vi "Master Program.vi"() -> ()   [LabVIEW 2017]
uses:
  <vilib>/Math Plots/3D Math Plots/3D Scatter/3D Scatter XCtrl/3D Scatter.xctl
  <vilib>/Math Plots/3D Math Plots/3D Comet/3D Comet XCtrl/3D Comet.xctl
  <vilib>/Math Plots/3D Math Plots/3D Surface/3D Surface XCtrl/3D Surface.xctl
  <vilib>/Instr/_visa.llb/VISA Flush IO Buffer Mask.ctl
  Globals.vi
  <vilib>/Instr/_visa.llb/VISA Configure Serial Port (Instr).vi
  <vilib>/Math Plots/3D Math Plots/3D Scatter/3D Scatter Datatype/Public/Plot Helper (Vector).vi
  <vilib>/Math Plots/3D Math Plots/3D Comet/3D Comet Datatype/Public/Plot Helper (Vector).vi
  <vilib>/Utility/file.llb/Read Delimited Spreadsheet (DBL).vi
  <vilib>/Utility/cursorutil.llb/Set Cursor (Icon Pict).vi
  <vilib>/Math Plots/3D Math Plots/3D Comet/3D Comet Datatype/3D Comet Datatype.lvclass
  <vilib>/Math Plots/3D Math Plots/3D Scatter/3D Scatter Datatype/3D Scatter Datatype.lvclass
  <vilib>/FTP/NI_FTP.lvlib
panel:
  out "error out 6":errorcluster caption="error out"
  out "error out 5":errorcluster
  out "file error":errorcluster
  out "error out 4":errorcluster
  out "state":dbl
  out "VISA resource name out":refnum<visa-resource-name>
  out "error out 3":errorcluster caption="error out"
  out "error out 2":errorcluster
  out "error out":errorcluster
  out "Message Window":string
  out "Data load indicator":bool
  in  "stop":bool
  in  "Close Figures":bool
  out "Load":string
  out "NX path":path caption="selected path"
  in  "Tab Control":T1(tab)
  in  "Open Webcam":bool
  in  "Form Type":u16(ring) items=["Pyramid", "NX Pattern"]
  in  "Save":bool
  out "Calculated Depth":dbl
  in  "vangle":dbl
  in  "overlap":dbl
  in  "increment":dbl
  in  "width":dbl
  in  "layers":dbl
  in  "height":dbl
  in  "Min_dist":dbl
  out "3D Scatter 2":refnum<class "3D Plot Datatype.lvclass">[](xcontrol)
  out "3D Comet":refnum<class "3D Plot Datatype.lvclass">[](xcontrol)
  in  "refresh":bool
  in  "interpolate":bool
  in  "Upload Path":bool
  in  "z offset":dbl
  in  "y offset":dbl
  in  "x offset":dbl
  in  "Min_dist initial":dbl
  in  "height initial":dbl
  in  "layers initial":dbl
  in  "width initial":dbl
  in  "increment initial":dbl
  in  "overlap initial":dbl
  in  "vangle initial":dbl
  out "Calculated Depth initial":dbl
  in  "Save Initial":bool
  out "3D Comet 2":refnum<class "3D Plot Datatype.lvclass">[](xcontrol)
  in  "Spin Graph":dbl(knob) min=-2.0 max=2.0 step=0.25 scale=-2.0..2.0
  out "Normalized Error":dbl
  in  "Plot":bool
  in  "Figure":bool
  in  "Matlab Plot":u16(ring) items=["Reference", "Initial Form Path", "Measured Data", "Error vs. Iteration", "Error vs. Command", "Error Surface", "Current Correction Path", "Error vs. Translation", "Custom"]
  out "3D Comet 3":refnum<class "3D Plot Datatype.lvclass">[](xcontrol)
  out "3D Surface":refnum<class "3D Plot Datatype.lvclass">[](xcontrol)
  out "Correction #":dbl
  in  "Save Correction":bool
  in  "Correction Factor K":dbl(slide) min=0.0 max=1.0 step=0.01 scale=0.0..1.0
  in  "Load Final Data":bool
  in  "Load Initial":bool
  in  "Graph Select":u16(ring) items=["Error Plot", "Measured Data", "Path Plot", "Reference"]
  in  "Upload Path":bool
  in  "Graph Format Code":string
  in  "Stop Robot":bool
  out "Standby":bool=TRUE
  in  "Start Robot":bool
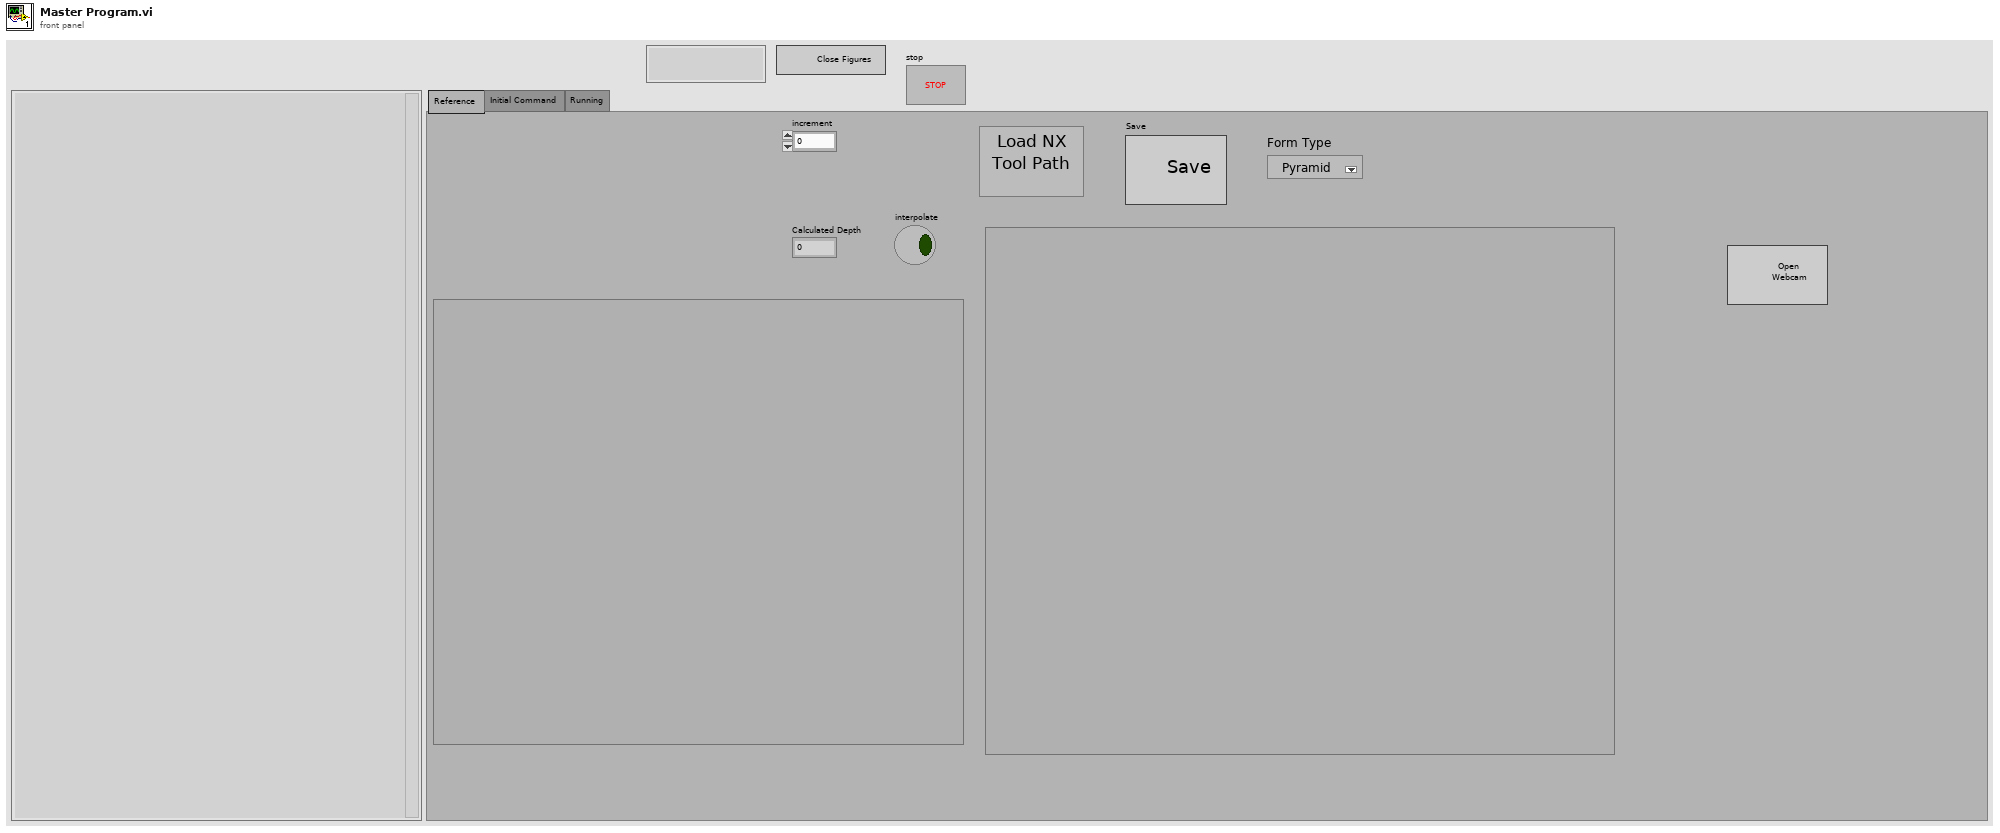
[diagram p1: front panel]
types:
  T1 = enum32{"Reference ", "Initial Command", "Running"}
  T2 = cluster{"x shift":dbl, "y shift":dbl, "z shift":dbl, "Theta x":dbl, "Theta y":dbl}
  T3 = cluster{"increment":dbl, "vangle":dbl, "overlap":dbl, "width":dbl, "height":dbl, "layers":dbl, "min_dist":dbl}
  T4 = cluster{"increment initial":dbl, "vangle initial":dbl, "overlap initial":dbl, "width initial":dbl, "height initial":dbl, "layers initial":dbl}
  T5 = typedef "VISA Flush IO Buffer Mask.ctl" = u16
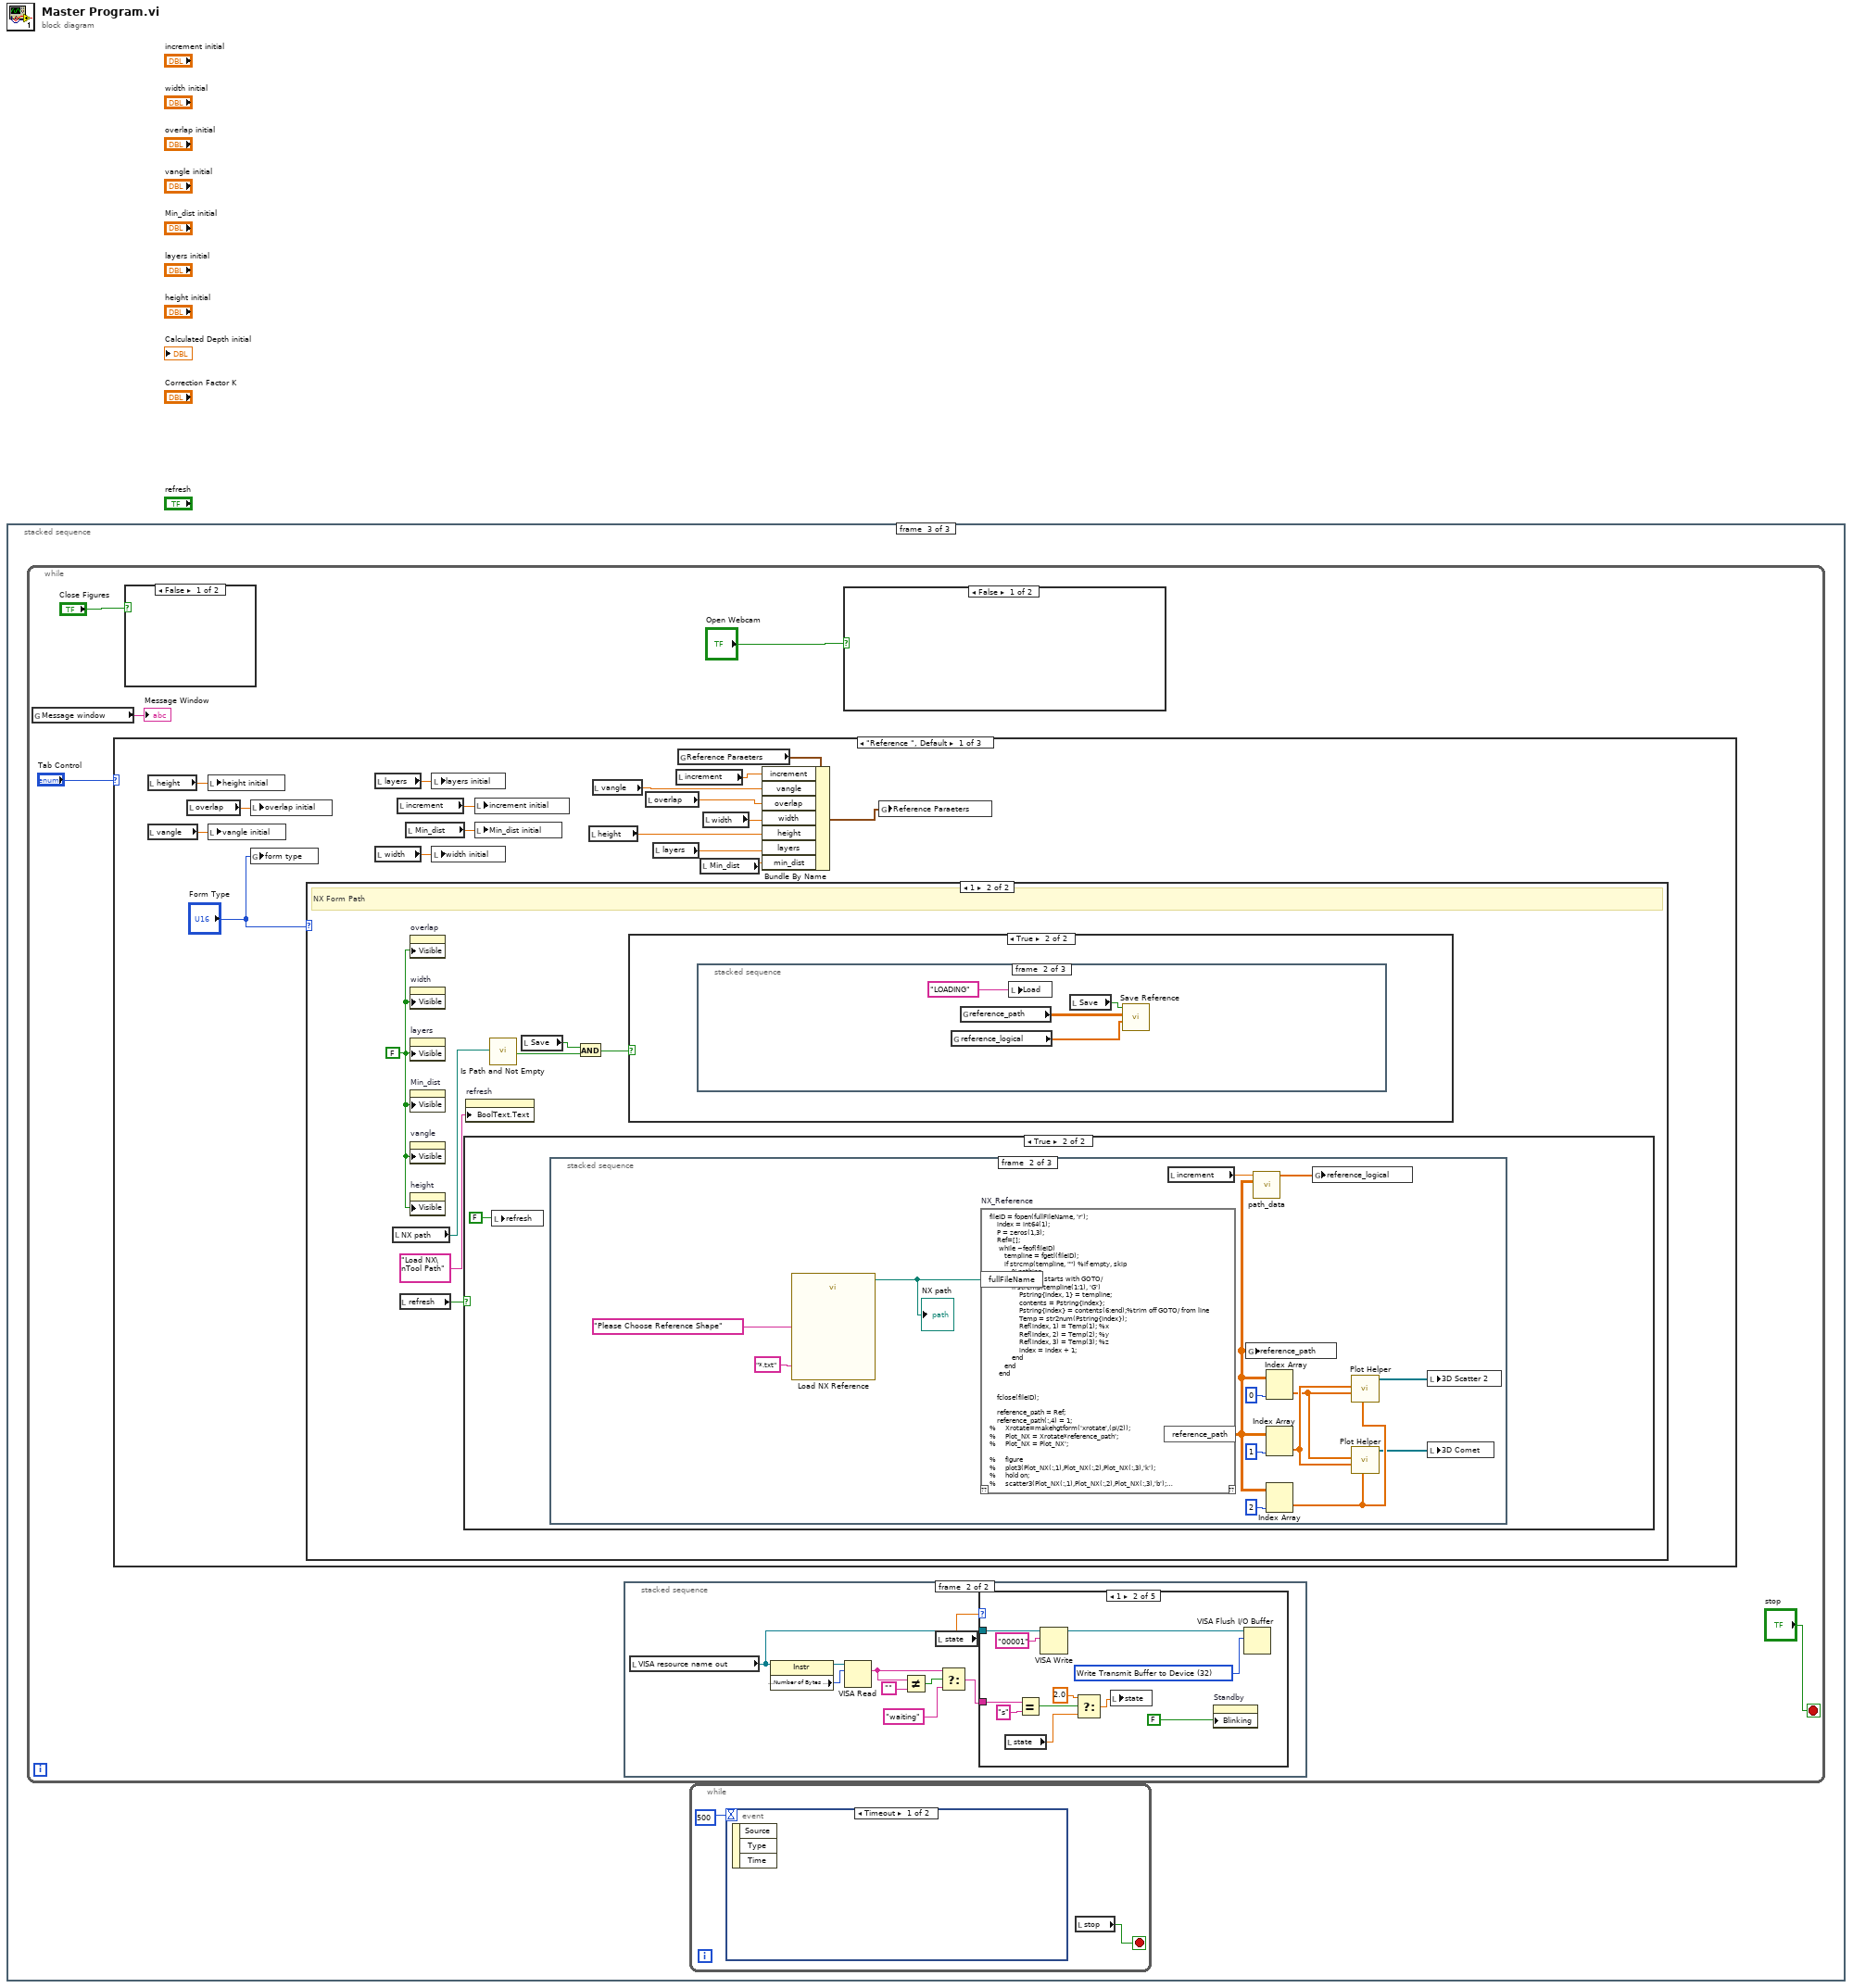
[diagram p0: block diagram]
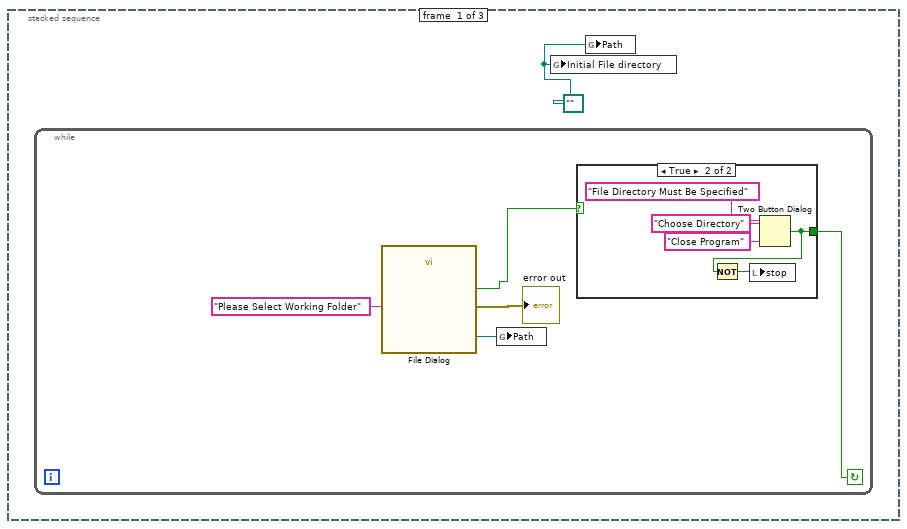
[diagram p2: hidden frame]
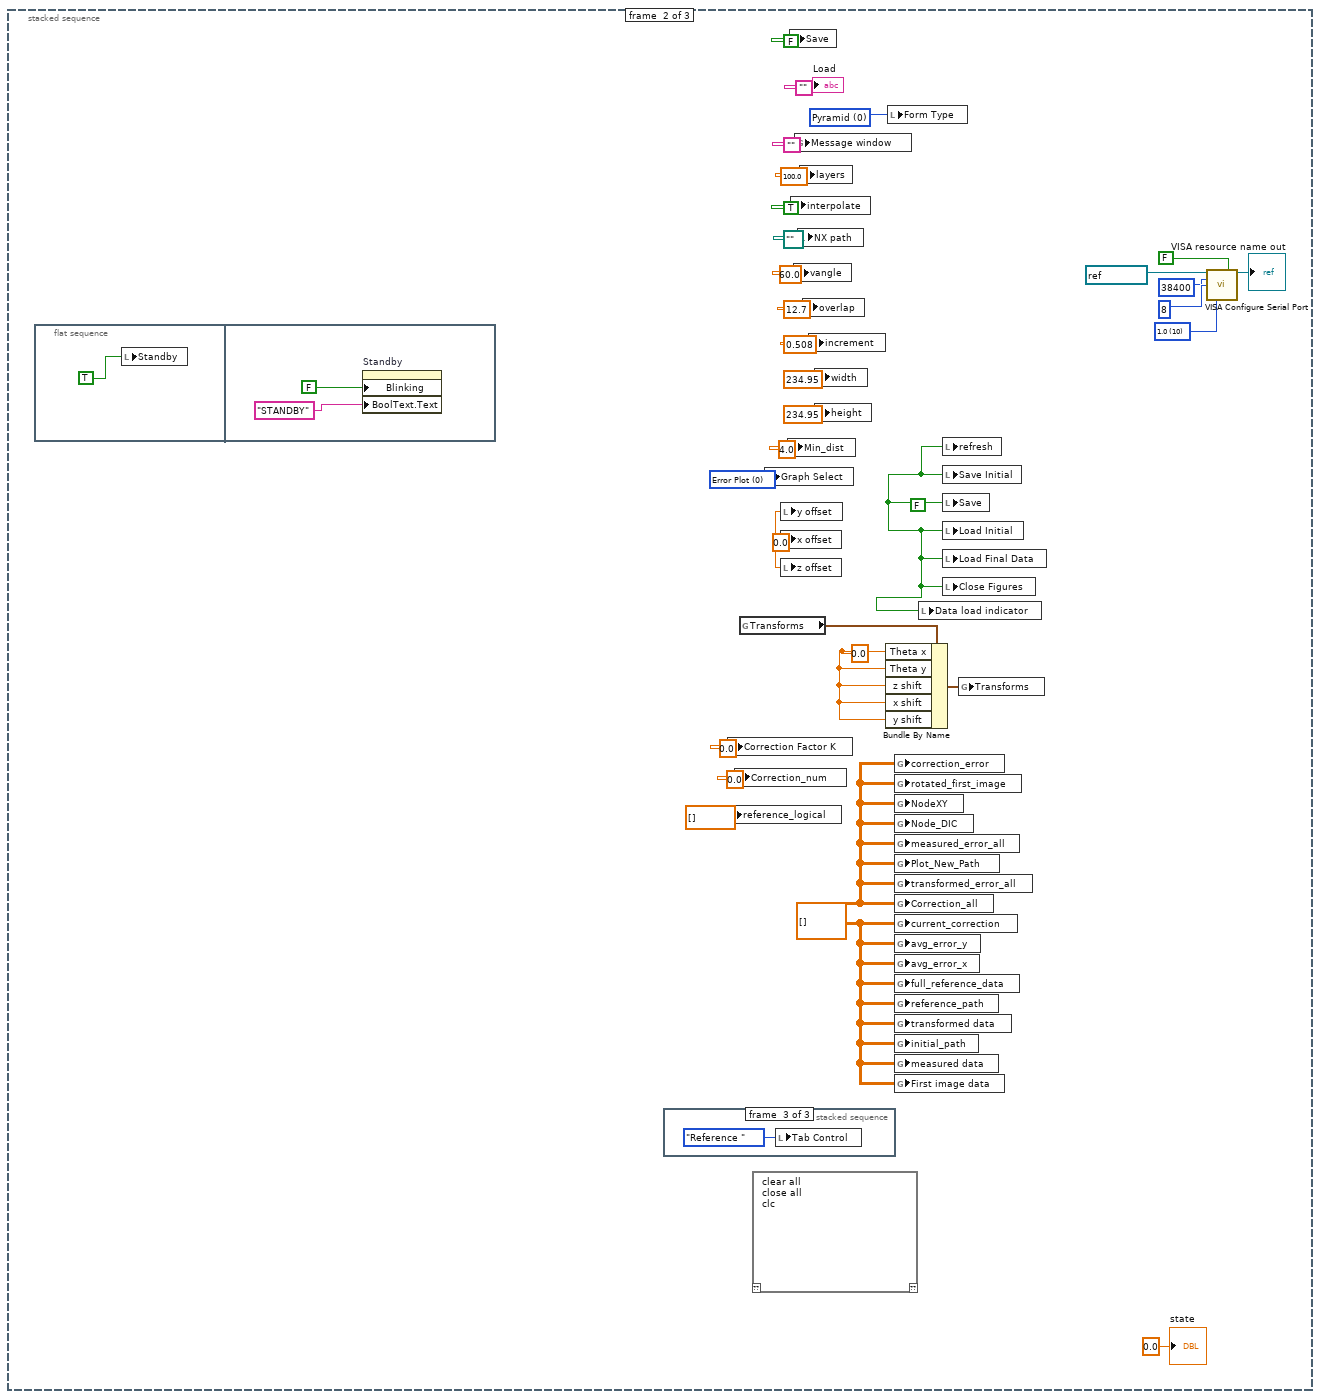
[diagram p4: hidden frame]
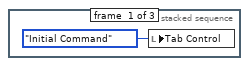
[diagram p5: hidden frame]
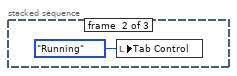
[diagram p6: hidden frame]
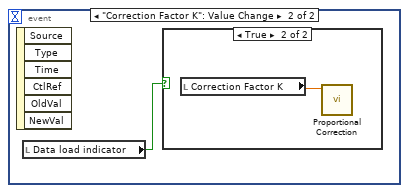
[diagram p7: hidden frame]
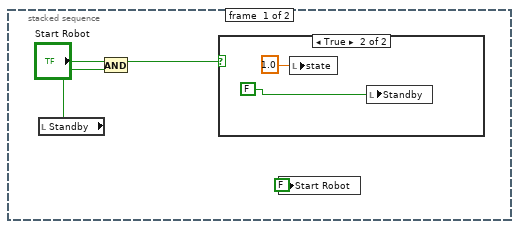
[diagram p9: hidden frame]
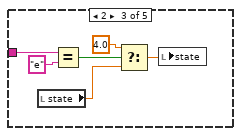
[diagram p12: hidden frame]
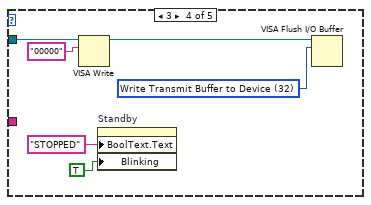
[diagram p13: hidden frame]
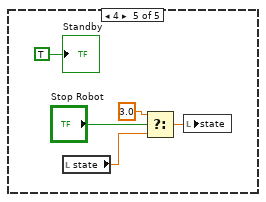
[diagram p14: hidden frame]
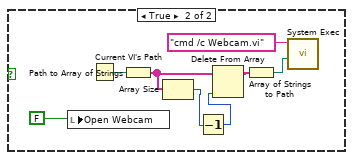
[diagram p15: hidden frame]
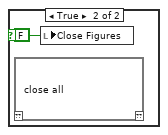
[diagram p16: hidden frame]
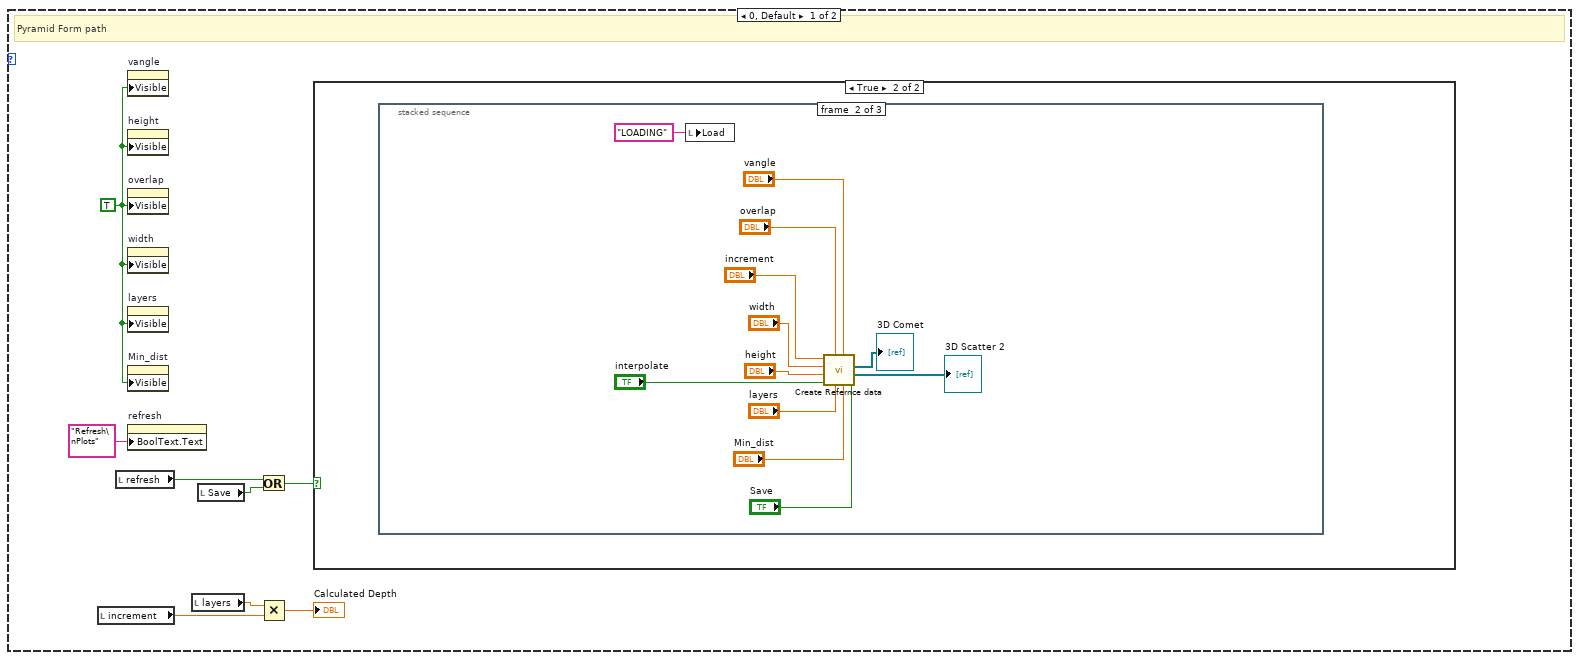
[diagram p17: hidden frame]
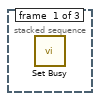
[diagram p19: hidden frame]
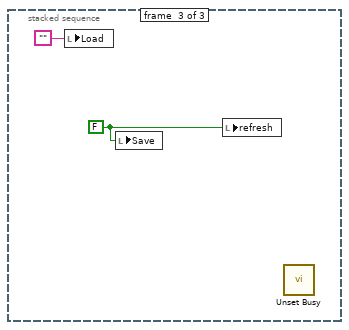
[diagram p20: hidden frame]
diagram:
  n1 = stacked-sequence {
    frame #0 {
      w1 = path "" ("Initial File directory")
      n2 = while {
        stop <- w2 continue-if-true
        n3 = call "File Dialog"("prompt"="Please Select Working Folder") -> ("selected path"=w4:path, "cancelled"=w3:bool, "error out"=→"error out":errorcluster)  [unwired: 11 in, 1 out]
        n4 = global write "Globals.vi" "Path"(w4) -> ()
        n5 = case shown="True" w3 {
          selector: w3 -> [w7 _]
          tunnel: [w7 w8] -> w2
          frame False {
          }
          frame True {
            n6 = Two Button Dialog(message="File Directory Must Be Specified", 1:"Close Program" ("F button name (\"Cancel\")"), 2:"Choose Directory" ("T button name (\"OK\")")) -> (T button?=w8:bool)
            n7 = Not(x=w8) -> (.not. x?=w9:bool)
            n8 = local write "stop"(w9) -> ()
          }
        }
      }
      n9 = global write "Globals.vi" "Initial File directory"(w1) -> ()
      n10 = global write "Globals.vi" "Path"(w1) -> ()
    }
    frame #1 {
      w16 = u16 10 items=["1.0"=10, "1.5"=15, "2.0"=20] ("stop bits (10: 1 bit)")
      w20 = u16 0 items=["Error Plot", "Measured Data", "Path Plot", "Reference"] ("Graph Select")
      w21 = dbl[][] []
      w25 = FALSE ("refresh")
      w26 = 0.0 ("z offset")
      w27 = 0.0
      w31 = u16 0 items=["Pyramid", "NX Pattern"] ("Form Type")
      n11 = flat-sequence {
        frame #0 {
          n12 = local write "Standby"(TRUE ("Standby")) -> ()
        }
        frame #1 {
          n13 = property on="Standby" class="Bool (strict)"("Blinking"=FALSE, "BoolText.Text"="STANDBY" ("Boolean Text.Text")) -> ()  [unwired: 2 in, 2 out]
        }
      }
      n14 = stacked-sequence {
        frame #0 {
          n15 = local write "Tab Control"(T1."Initial Command" ("Tab Control")) -> ()
        }
        frame #1 {
          n16 = local write "Tab Control"(T1."Running" ("Tab Control")) -> ()
        }
        frame #2 {
          n17 = local write "Tab Control"(T1."Reference " ("Tab Control")) -> ()
        }
      }
      n18 = global write "Globals.vi" "reference_logical"(dbl[] []) -> ()
      n19 = local write "Correction Factor K"(0.0 ("Correction Factor K")) -> ()
      n20 = global write "Globals.vi" "Correction_num"(0.0 ("Correction_num")) -> ()
      n21 = global read "Globals.vi" "Transforms"() -> (w29:T2)
      n22 = script code="clear all\nclose all\nclc"() -> ()  [unwired: 1 in, 1 out]
      n23 = local write "Graph Select"(w20) -> ()
      n24 = local write "y offset"(w26) -> ()
      n25 = local write "x offset"(w26) -> ()
      n26 = local write "z offset"(w26) -> ()
      n27 = local write "Min_dist"(4.0 ("vangle")) -> ()
      n28 = local write "Save"(FALSE ("Save Button")) -> ()
      n29 = local write "interpolate"(TRUE ("Interpolate")) -> ()
      n30 = local write "vangle"(60.0 ("vangle")) -> ()
      n31 = global write "Globals.vi" "Message window"("") -> ()
      n32 = local write "NX path"(path "" ("y")) -> ()
      n33 = local write "layers"(100.0 ("vangle")) -> ()
      n34 = local write "overlap"(12.7 ("vangle")) -> ()
      n35 = local write "increment"(0.508 ("vangle")) -> ()
      n36 = local write "width"(234.95 ("vangle")) -> ()
      n37 = local write "height"(234.95 ("vangle")) -> ()
      n38 = Bundle By Name(cluster=w29, "Theta x"=w27, "Theta y"=w27, "z shift"=w27, "x shift"=w27, "y shift"=w27) -> (w28:T2)
      n39 = local write "Form Type"(w31) -> ()
      n40 = global write "Globals.vi" "correction_error"(w21) -> ()
      n41 = global write "Globals.vi" "rotated_first_image"(w21) -> ()
      n42 = global write "Globals.vi" "NodeXY"(w21) -> ()
      n43 = global write "Globals.vi" "Node_DIC"(w21) -> ()
      n44 = global write "Globals.vi" "measured_error_all"(w21) -> ()
      n45 = global write "Globals.vi" "Plot_New_Path"(w21) -> ()
      n46 = global write "Globals.vi" "transformed_error_all"(w21) -> ()
      n47 = global write "Globals.vi" "Correction_all"(w21) -> ()
      n48 = global write "Globals.vi" "current_correction"(w21) -> ()
      n49 = global write "Globals.vi" "avg_error_y"(w21) -> ()
      n50 = global write "Globals.vi" "avg_error_x"(w21) -> ()
      n51 = global write "Globals.vi" "full_reference_data"(w21) -> ()
      n52 = global write "Globals.vi" "reference_path"(w21) -> ()
      n53 = global write "Globals.vi" "transformed data"(w21) -> ()
      n54 = global write "Globals.vi" "initial_path"(w21) -> ()
      n55 = global write "Globals.vi" "measured data"(w21) -> ()
      n56 = global write "Globals.vi" "First image data"(w21) -> ()
      n57 = local write "Data load indicator"(w25) -> ()
      n58 = local write "refresh"(w25) -> ()
      n59 = local write "Save Initial"(w25) -> ()
      n60 = local write "Save"(w25) -> ()
      n61 = local write "Load Initial"(w25) -> ()
      n62 = local write "Load Final Data"(w25) -> ()
      n63 = local write "Close Figures"(w25) -> ()
      n64 = global write "Globals.vi" "Transforms"(w28) -> ()
      n65 = call-poly "VISA Configure Serial Port"("VISA resource name"=refnum<visa-resource-name> "COM2", "Enable Termination\nChar (T)"=FALSE ("Enable Termination\nChar (T)"), "baud rate (9600)"=u32 38400, "data bits (8)"=u16 8, "stop bits (10: 1 bit)"=w16) -> ("VISA resource name out"=→"VISA resource name out":refnum<visa-resource-name>)  [unwired: 9 in, 1 out]
      "Load" <- ""
      "state" <- 0.0 ("state")
    }
    frame #2 {
      n66 = while {
        stop <- "stop" stop-if-true
        n67 = global read "Globals.vi" "Message window"() -> (→"Message Window":string)
        n68 = case shown="\"Reference \", Default" "Tab Control" {
          frame "Reference ", Default {
            n69 = local read "height"() -> (w122:dbl)
            n70 = local read "vangle"() -> (w123:dbl)
            n71 = local read "overlap"() -> (w119:dbl)
            n72 = local write "height initial"(w122) -> ()
            n73 = local write "vangle initial"(w123) -> ()
            n74 = local write "overlap initial"(w119) -> ()
            n75 = global write "Globals.vi" "form type"("Form Type") -> ()
            n76 = case shown="1" "Form Type" {
              frame 0, Default {
                w128 = TRUE
                # "Pyramid Form path"
                n77 = local read "increment"() -> (w129:dbl)
                n78 = local read "refresh"() -> (w134:bool)
                n79 = property on="vangle" class="DigNum (strict)"("Visible"=w128) -> ()  [unwired: 2 in, 2 out]
                n80 = property on="height" class="DigNum (strict)"("Visible"=w128) -> ()  [unwired: 2 in, 2 out]
                n81 = property on="overlap" class="DigNum (strict)"("Visible"=w128) -> ()  [unwired: 2 in, 2 out]
                n82 = property on="width" class="DigNum (strict)"("Visible"=w128) -> ()  [unwired: 2 in, 2 out]
                n83 = property on="layers" class="DigNum (strict)"("Visible"=w128) -> ()  [unwired: 2 in, 2 out]
                n84 = property on="Min_dist" class="DigNum (strict)"("Visible"=w128) -> ()  [unwired: 2 in, 2 out]
                n85 = property on="refresh" class="Bool (strict)"("BoolText.Text"="Refresh\nPlots" ("Boolean Text.Text")) -> ()  [unwired: 2 in, 2 out]
                n86 = local read "layers"() -> (w130:dbl)
                n87 = local read "Save"() -> (w133:bool)
                n88 = Or(x=w134, y=w133) -> (x .or. y?=w132:bool)
                n89 = Multiply(x=w130, y=w129) -> (x*y=→"Calculated Depth":dbl)
                n90 = case shown="True" w132 {
                  frame False {
                  }
                  frame True {
                    n91 = stacked-sequence {
                      frame #0 {
                        n92 = call <vilib>:"Set Busy.vi"() -> ()  [unwired: 10 in, 2 out]
                      }
                      frame #1 {
                        n93 = local write "Load"("LOADING") -> ()
                        n94 = call "Create Refernce data.vi"("Save Button"="Save", "Min_dist"="Min_dist", "vangle"="vangle", "layers"="layers", "overlap"="overlap", "Interpolate"="interpolate", "height"="height", "width"="width", "increment"="increment") -> ("Reference"=→"3D Scatter 2":refnum<class "3D Plot Datatype.lvclass">[], "3D Comet"=→"3D Comet":refnum<class "3D Plot Datatype.lvclass">[])  [unwired: 1 in]
                      }
                      frame #2 {
                        w148 = FALSE ("Save Button")
                        n95 = local write "Load"("") -> ()
                        n96 = local write "Save"(w148) -> ()
                        n97 = local write "refresh"(w148) -> ()
                        n98 = call <vilib>:"Unset Busy.vi"() -> ()  [unwired: 11 in, 1 out]
                      }
                    }
                  }
                }
              }
              frame 1 {
                w155 = FALSE
                # "NX Form Path"
                n99 = local read "NX path"() -> (w149:path)
                n100 = local read "refresh"() -> (w154:bool)
                n101 = property on="overlap" class="DigNum (strict)"("Visible"=w155) -> ()  [unwired: 2 in, 2 out]
                n102 = property on="width" class="DigNum (strict)"("Visible"=w155) -> ()  [unwired: 2 in, 2 out]
                n103 = property on="layers" class="DigNum (strict)"("Visible"=w155) -> ()  [unwired: 2 in, 2 out]
                n104 = property on="Min_dist" class="DigNum (strict)"("Visible"=w155) -> ()  [unwired: 2 in, 2 out]
                n105 = property on="vangle" class="DigNum (strict)"("Visible"=w155) -> ()  [unwired: 2 in, 2 out]
                n106 = property on="height" class="DigNum (strict)"("Visible"=w155) -> ()  [unwired: 2 in, 2 out]
                n107 = case shown="True" w154 {
                  frame False {
                  }
                  frame True {
                    n108 = local write "refresh"(FALSE ("refresh")) -> ()
                    n109 = stacked-sequence {
                      frame #0 {
                        n110 = local write "Load"("LOADING") -> ()
                        n111 = call <vilib>:"Set Busy.vi"() -> ()  [unwired: 10 in, 2 out]
                      }
                      frame #1 {
                        n112 = call "Load NX Reference"("prompt"="Please Choose Reference Shape", "pattern (all files)"="*.txt") -> ("selected path"=w177:path)  [unwired: 10 in, 3 out]
                        "NX path" <- w177
                        n113 = script code="fileID = fopen(fullFileName, 'r');\n    index = int64(1);\n    P = zeros(1,3);\n    Ref=[];\n     while ~feof(fileID)\t\n        templine = fgetl(fileID);\n        if strcmp(templine, \"\") %if empty, skip\n            %nothing\n        else %if line starts with GOTO/\n            if strcmp(templine(1:1), 'G')\n                Pstring{index, 1} = templine;\n                contents = Pstring{index};\n                Pstring{index} = contents(6:end);%trim off GOTO/ from line\n                Temp = str2num(Pstring{index});\n                Ref(index, 1) = Temp(1); %x\n                Ref(index, 2) = Temp(2); %y\n                Ref(index, 3) = Temp(3); %z\n                index = index + 1; \n            end\n        end\n     end\n \n\n    fclose(fileID);\n    \n    reference_path = Ref;\n    reference_path(:,4) = 1;\n%     Xrotate=makehgtform('xrotate',(pi/2));\n%     Plot_NX = Xrotate*reference_path';\n%     Plot_NX = Plot_NX';\n\n%     figure\n%     plot3(Plot_NX(:,1),Plot_NX(:,2),Plot_NX(:,3),'k');\n%     hold on;\n%     scatter3(Plot_NX(:,1),Plot_NX(:,2),Plot_NX(:,3),'b');\n%     hold off;\n   \n%     xlabel(\"X (mm)\");\n%     ylabel(\"Z (mm)\");\n%     zlabel(\"Y (mm)\");\n%     \n    reference_path = reference_path(:,1:3);" "NX_Reference"("fullFileName"=w177) -> ("reference_path"=w171:dbl[][])  [unwired: 1 in, 1 out]
                        n114 = local read "increment"() -> (w176:dbl)
                        n115 = global write "Globals.vi" "reference_path"(w171) -> ()
                        n116 = call "path_data.vi"("path in"=w171, "increment"=w176) -> ("path logical"=w175:dbl[])  [unwired: 9 in]
                        n117 = Index Array(array=w171, index (col)=0 ("index")) -> (element=w169:dbl[])  [unwired: 1 in]
                        n118 = Index Array(array=w171, index (col)=1 ("index")) -> (element=w170:dbl[])  [unwired: 1 in]
                        n119 = Index Array(array=w171, index (col)=2 ("index")) -> (element=w168:dbl[])  [unwired: 1 in]
                        n120 = global write "Globals.vi" "reference_logical"(w175) -> ()
                        n121 = call-poly <vilib>:"Plot Helper.vi"("z vector"=w168, "y vector"=w169, "x vector"=w170) -> ("3D Plot lvclass Array out"=w166:refnum<class "3D Plot Datatype.lvclass">[])  [unwired: 3 in, 5 out]
                        n122 = call-poly <vilib>:"Plot Helper.vi"("z vector"=w168, "y vector"=w170, "x vector"=w169) -> ("3D Plot lvclass Array out"=w167:refnum<class "3D Plot Datatype.lvclass">[])  [unwired: 3 in, 5 out]
                        n123 = local write "3D Scatter 2"(w166) -> ()
                        n124 = local write "3D Comet"(w167) -> ()
                      }
                      frame #2 {
                        n125 = local write "Load"("") -> ()
                        n126 = call <vilib>:"Unset Busy.vi"() -> ()  [unwired: 11 in, 1 out]
                      }
                    }
                  }
                }
                n127 = property on="refresh" class="Bool (strict)"("BoolText.Text"="Load NX\nTool Path" ("Boolean Text.Text")) -> ()  [unwired: 2 in, 2 out]
                n128 = call <vilib>:"Is Path and Not Empty.vi"("path"=w149) -> ("Is Path and Not Empty?"=w150:bool)  [unwired: 4 in]
                n129 = local read "Save"() -> (w151:bool)
                n130 = And(x=w151, y=w150) -> (x .and. y?=w152:bool)
                n131 = case shown="True" w152 {
                  frame False {
                    n132 = local write "Save"(FALSE ("Save")) -> ()
                  }
                  frame True {
                    n133 = stacked-sequence {
                      frame #0 {
                        n134 = call <vilib>:"Set Busy.vi"() -> ()  [unwired: 10 in, 2 out]
                      }
                      frame #1 {
                        n135 = global read "Globals.vi" "reference_logical"() -> (w159:dbl[])
                        n136 = global read "Globals.vi" "reference_path"() -> (w160:dbl[][])
                        n137 = local write "Load"("LOADING") -> ()
                        n138 = local read "Save"() -> (w158:bool)
                        n139 = call "Save Reference.vi"("Refernce_logical"=w159, "Reference path"=w160, "Save Button"=w158) -> ()  [unwired: 9 in]
                      }
                      frame #2 {
                        n140 = local write "Save"(FALSE ("Save")) -> ()
                        n141 = local write "Load"("") -> ()
                        n142 = call <vilib>:"Unset Busy.vi"() -> ()  [unwired: 11 in, 1 out]
                      }
                    }
                  }
                }
              }
            }
            n143 = local read "layers"() -> (w125:dbl)
            n144 = local read "width"() -> (w121:dbl)
            n145 = local read "increment"() -> (w120:dbl)
            n146 = local read "Min_dist"() -> (w124:dbl)
            n147 = local write "layers initial"(w125) -> ()
            n148 = local write "width initial"(w121) -> ()
            n149 = local write "increment initial"(w120) -> ()
            n150 = local write "Min_dist initial"(w124) -> ()
            n151 = local read "height"() -> (w115:dbl)
            n152 = local read "vangle"() -> (w116:dbl)
            n153 = local read "overlap"() -> (w113:dbl)
            n154 = local read "layers"() -> (w110:dbl)
            n155 = local read "increment"() -> (w112:dbl)
            n156 = global read "Globals.vi" "Reference Paraeters"() -> (w118:T3)
            n157 = local read "Min_dist"() -> (w111:dbl)
            n158 = local read "width"() -> (w114:dbl)
            n159 = Bundle By Name(cluster=w118, "increment"=w112, "vangle"=w116, "overlap"=w113, "width"=w114, "height"=w115, "layers"=w110, "min_dist"=w111) -> (w117:T3)
            n160 = global write "Globals.vi" "Reference Paraeters"(w117) -> ()
          }
          frame "Initial Command" {
            n161 = global read "Globals.vi" "form type"() -> (w181:u16)
            n162 = case shown="True" "Upload Path" {
              frame False {
              }
              frame True {
                n163 = local write "Upload Path"(FALSE) -> ()
                n164 = call "File Dialog5"("prompt"="Select Initial Form Path", "pattern (all files)"="*.csv") -> ("selected path"=w185:path, "cancelled"=w184:bool, "error out"=→"error out 6":errorcluster)  [unwired: 10 in, 1 out]
                n165 = case shown="False" w184 {
                  tunnel: w185 -> [w218 _]
                  frame False {
                    n166 = call-poly <vilib>:"Read Delimited Spreadsheet.vi"("file path (dialog if empty)"=w218, "format (%.3f)"="%.5f", "delimiter (\\t)"="," ("delimiter (\\t)")) -> ("all rows"=w221:dbl[][], "first row"=w224:dbl[])  [unwired: 7 in, 4 out]
                    n167 = Array Max & Min(array=w224) -> (max value=w222:dbl, min value=w223:dbl)  [unwired: 2 out]
                    n168 = Equal?(x=w222, y=w223) -> (x = y?=w220:bool)
                    n169 = case shown="False" w220 {
                      tunnel: w221 -> [w226 w229]
                      tunnel: [w226 w227] -> w196
                      frame False {
                      }
                      frame True {
                        n170 = Delete From Array(array=w229, index (row)=0) -> (array with subset deleted=w227:dbl[][])  [unwired: 2 in, 1 out]
                      }
                    }
                    n171 = local read "x offset"() -> (w195:dbl)
                    n172 = local read "y offset"() -> (w194:dbl)
                    n173 = local read "z offset"() -> (w193:dbl)
                    n174 = script code="% Apply user's translations in x, y, and z\n    xyz_translate = [1 0 0 xoffset; 0 1 0 yoffset; 0 0 1 zoffset; 0 0 0 1];\n    initial_corners(:,4) = 1;\n    initial_corners = xyz_translate*initial_corners';\n    initial_corners = initial_corners';" "apply offsets to corners"("initial_corners"=w196, "yoffset"=w194, "zoffset"=w193, "xoffset"=w195) -> ("initial_corners"=w215:dbl[][])  [unwired: 1 in, 1 out]
                    n175 = Delete From Array(array=w215, index (col)=3 ("disabled index (col)")) -> (array with subset deleted=w216:dbl[][])  [unwired: 2 in, 1 out]
                    n176 = Index Array(array=w215, index (col)=0 ("disabled index (col)")) -> (element=w212:dbl[])  [unwired: 1 in]
                    n177 = Index Array(array=w215, index (col)=1 ("disabled index (col)")) -> (element=w213:dbl[])  [unwired: 1 in]
                    n178 = Index Array(array=w215, index (col)=2 ("disabled index (col)")) -> (element=w214:dbl[])  [unwired: 1 in]
                    n179 = Current VI's Path() -> (path=w209:path)
                    n180 = global write "Globals.vi" "initial_path"(w216) -> ()
                    n181 = Path to Array of Strings(0:w209) -> (2:w210:string[])  [unwired: 1 out]
                    n182 = call-poly <vilib>:"Plot Helper.vi"("z vector"=w214, "y vector"=w213, "x vector"=w212) -> ("3D Plot lvclass Array out"=w188:refnum<class "3D Plot Datatype.lvclass">[])  [unwired: 3 in, 5 out]
                    n183 = call "path_data.vi"("path in"=w216, "increment"=1.0) -> ("path logical"=w217:dbl[])  [unwired: 9 in]
                    n184 = Array Size(array=w210) -> (size(s)=w207:i32)
                    n185 = global write "Globals.vi" "initial_logical"(w217) -> ()
                    n186 = local read "x offset"() -> (w191:dbl)
                    n187 = local read "y offset"() -> (w190:dbl)
                    n188 = local read "z offset"() -> (w189:dbl)
                    n189 = Decrement(x=w207) -> (x-1=w206:i32)
                    n190 = global read "Globals.vi" "Message window"() -> (w204:string)
                    n191 = Delete From Array(array=w210, index=w206) -> (array with subset deleted=w208:string[])  [unwired: 1 in, 1 out]
                    n192 = local write "3D Comet 2"(w188) -> ()
                    n193 = global read "Globals.vi" "form type"() -> (w192:u16)
                    n194 = Array of Strings to Path(0:w208) -> (2:w205:path)  [unwired: 1 in]
                    n195 = global read "Globals.vi" "Path"() -> (w203:path)
                    n196 = Path To String(path=w205) -> (string=w211:string)
                    n197 = call "Save Initial Command.vi"("Message window"=w204, "Directory"=w211, "Initial Path"=w215, "Path"=w203, "z offset"=w189, "y offset"=w190, "x offset"=w191, "form type"=w192) -> ("Window Output"=w202:string)  [unwired: 3 in]
                    n198 = global write "Globals.vi" "Message window"(w202) -> ()
                  }
                  frame True {
                  }
                }
              }
            }
            n199 = case shown="1" w181 {
              frame 0, Default {
                # "Pyramid form"
                n200 = local read "increment initial"() -> (w230:dbl)
                n201 = local read "layers initial"() -> (w231:dbl)
                n202 = case shown="True" "Save Initial" {
                  frame False {
                  }
                  frame True {
                    n203 = stacked-sequence {
                      frame #0 {
                        n204 = global read "Globals.vi" "initial command"() -> (w241:T4)
                        n205 = local read "increment initial"() -> (w239:dbl)
                        n206 = local read "overlap initial"() -> (w237:dbl)
                        n207 = local read "vangle initial"() -> (w238:dbl)
                        n208 = local read "height initial"() -> (w235:dbl)
                        n209 = local read "width initial"() -> (w236:dbl)
                        n210 = local read "layers initial"() -> (w234:dbl)
                        n211 = Bundle By Name(cluster=w241, "increment initial"=w239, "vangle initial"=w238, "overlap initial"=w237, "width initial"=w236, "height initial"=w235, "layers initial"=w234) -> (w240:T4)
                        n212 = call <vilib>:"Set Busy.vi"() -> ()  [unwired: 10 in, 2 out]
                        n213 = global write "Globals.vi" "initial command"(w240) -> ()
                      }
                      frame #1 {
                        n214 = local read "increment initial"() -> (w252:dbl)
                        n215 = local read "overlap initial"() -> (w243:dbl)
                        n216 = local read "vangle initial"() -> (w253:dbl)
                        n217 = local read "height initial"() -> (w245:dbl)
                        n218 = local read "width initial"() -> (w244:dbl)
                        n219 = local read "layers initial"() -> (w246:dbl)
                        n220 = local write "Load"("LOADING PATH") -> ()
                        n221 = call "Pyramid_Path.vi"("layers"=w246, "height"=w245, "vangle"=w253, "width"=w244, "increment"=w252, "overlap"=w243) -> ("reference_corners"=w251:dbl[][])  [unwired: 5 in]
                        n222 = call "Pyramid Initial Command.vi"("y offset"="y offset", "z offset"="z offset", "x offset"="x offset", "reference_corners"=w251, "increment initial"=w252) -> ("3D Comet 2"=→"3D Comet 2":refnum<class "3D Plot Datatype.lvclass">[])  [unwired: 6 in]
                      }
                      frame #2 {
                        n223 = local write "Save Initial"(FALSE) -> ()
                        n224 = local write "Load"("") -> ()
                        n225 = call <vilib>:"Unset Busy.vi"() -> ()  [unwired: 11 in, 1 out]
                      }
                    }
                  }
                }
                n226 = Multiply(x=w230, y=w231) -> (x*y=w232:dbl)
                n227 = local write "Calculated Depth initial"(w232) -> ()
              }
              frame 1 {
                # "NX Path"
                n228 = local read "Save Initial"() -> (w256:bool)
                n229 = case shown="True" w256 {
                  frame False {
                  }
                  frame True {
                    n230 = local write "Save Initial"(FALSE) -> ()
                    n231 = call "File Dialog2"("prompt"="Load Initial NX Tool Path", "pattern (all files)"="*.txt" ("pattern label")) -> ("selected path"=w257:path)  [unwired: 10 in, 3 out]
                    n232 = stacked-sequence {
                      tunnel: w257 -> [_ w266 _]
                      frame #0 {
                        n233 = call <vilib>:"Set Busy.vi"() -> ()  [unwired: 10 in, 2 out]
                        n234 = local write "Load"("LOADING") -> ()
                      }
                      frame #1 {
                        n235 = local read "y offset"() -> (w265:dbl)
                        n236 = local read "x offset"() -> (w264:dbl)
                        n237 = local read "z offset"() -> (w263:dbl)
                        n238 = call "NX Initial Command.vi"("z offset"=w263, "x offset"=w264, "y offset"=w265, "selected path"=w266) -> ("3D comet"=w262:refnum<class "3D Plot Datatype.lvclass">[])  [unwired: 1 in]
                        n239 = local write "3D Comet 2"(w262) -> ()
                      }
                      frame #2 {
                        n240 = call <vilib>:"Unset Busy.vi"() -> ()  [unwired: 11 in, 1 out]
                        n241 = local write "Load"("") -> ()
                      }
                    }
                  }
                }
              }
            }
          }
          frame "Running" {
            n242 = global read "Globals.vi" "Correction_num"() -> (→"Correction #":dbl)
            n243 = global read "Globals.vi" "Transforms"() -> (w292:T2)
            n244 = feedback-in #1("Graph Select") -> ()
            n245 = feedback #1() -> (w279:u16)  [unwired: 1 in]
            n246 = case shown="True" "Load Initial" {
              frame False {
              }
              frame True {
                n247 = local write "Load Initial"(FALSE ("Load Initial")) -> ()
                n248 = call "File Dialog3"("prompt"="Select Reference Data", "pattern (all files)"="*.csv") -> ("selected path"=w386:path, "cancelled"=w384:bool, "error out"=→"error out 3":errorcluster)  [unwired: 10 in, 1 out]
                n249 = case shown="False" w384 {
                  tunnel: w386 -> [w390 _]
                  frame False {
                    n250 = call-poly <vilib>:"Read Delimited Spreadsheet.vi"("file path (dialog if empty)"=w390, "format (%.3f)"="%.5f", "delimiter (\\t)"="," ("delimiter (\\t)")) -> ("all rows"=w393:dbl[][], "first row"=w396:dbl[])  [unwired: 7 in, 4 out]
                    n251 = Array Max & Min(array=w396) -> (max value=w394:dbl, min value=w395:dbl)  [unwired: 2 out]
                    n252 = Equal?(x=w394, y=w395) -> (x = y?=w392:bool)
                    n253 = case shown="False" w392 {
                      tunnel: w393 -> [w398 w401]
                      tunnel: [w398 w399] -> w389
                      frame False {
                      }
                      frame True {
                        n254 = Delete From Array(array=w401, index (row)=0) -> (array with subset deleted=w399:dbl[][])  [unwired: 2 in, 1 out]
                      }
                    }
                    n255 = call "Calculate Transform.vi"("all rows"=w389) -> ()  [unwired: 11 in]
                  }
                  frame True {
                  }
                }
              }
            }
            n256 = Not Equal?(x="Graph Select", y=w279) -> (x != y?=w278:bool)
            n257 = Unbundle By Name(w292) -> ("x shift"=w291:dbl, "y shift"=w290:dbl, "z shift"=w289:dbl, "Theta x"=w288:dbl, "Theta y"=w287:dbl)
            n258 = stacked-sequence {
              tunnel: "Graph Select" -> [w327 w334]
              tunnel: w278 -> [w326 w339]
              frame #0 {
                n259 = case shown="True" w326 {
                  tunnel: w327 -> [_ w328]
                  frame False {
                  }
                  frame True {
                    n260 = case shown="2" w328 {
                      frame 0, Default {
                        w329 = TRUE
                        n261 = property on="3D Surface" class="3D Surface (strict)"("Visible"=w329) -> ()  [unwired: 2 in, 2 out]
                        n262 = Not(x=w329) -> (.not. x?=w330:bool)
                        n263 = property on="3D Comet 3" class="3D Comet (strict)"("Visible"=w330) -> ()  [unwired: 2 in, 2 out]
                      }
                      frame 2 {
                        w331 = FALSE
                        n264 = property on="3D Surface" class="3D Surface (strict)"("Visible"=w331) -> ()  [unwired: 2 in, 2 out]
                        n265 = Not(x=w331) -> (.not. x?=w332:bool)
                        n266 = property on="3D Comet 3" class="3D Comet (strict)"("Visible"=w332) -> ()  [unwired: 2 in, 2 out]
                      }
                    }
                  }
                }
              }
              frame #1 {
                n267 = global read "Globals.vi" "Correction_num"() -> (w340:dbl)
                n268 = Not Equal?(x=w334, y=u16 0) -> (x != y?=w335:bool)
                n269 = Not Equal To 0?(x=w340) -> (x != 0?=w337:bool)
                n270 = Or(x=w337, y=w335) -> (x .or. y?=w336:bool)
                n271 = And(x=w336, y=w339) -> (x .and. y?=w338:bool)
                n272 = case shown="True" w338 {
                  tunnel: w334 -> [_ w341]
                  frame False {
                  }
                  frame True {
                    n273 = call "Labview Plots.vi"("3d Graph Selector"=w341) -> ("surface"=→"3D Surface":refnum<class "3D Plot Datatype.lvclass">[], "comet"=→"3D Comet 3":refnum<class "3D Plot Datatype.lvclass">[])  [unwired: 8 in]
                  }
                }
              }
            }
            n274 = Compound Arithmetic op=ADD(w291, w290, w289, w288, w287) -> (w286:dbl)
            n275 = Not Equal?(x=w286, y=0.0) -> (x != y?=w284:bool)
            n276 = And(x="Load Final Data", y=w284) -> (x .and. y?=w282:bool)
            n277 = case shown="True" w282 {
              frame False {
              }
              frame True {
                n278 = stacked-sequence {
                  seq-local: [w348 _ _ _] -> [_ w365 w370 w373]
                  frame #0 {
                    n279 = call "File Dialog4"("prompt"="Select Final Data", "pattern (all files)"="*.csv") -> ("selected path"=w351:path, "cancelled"=w348:bool)  [unwired: 10 in, 2 out]
                    n280 = case shown="False" w348 {
                      tunnel: w351 -> [w360 _]
                      frame False {
                        n281 = call-poly <vilib>:"Read Delimited Spreadsheet.vi"("file path (dialog if empty)"=w360, "format (%.3f)"="%.5f", "delimiter (\\t)"="," ("delimiter (\\t)")) -> ("all rows"=w357:dbl[][], "first row"=w354:dbl[])  [unwired: 7 in, 4 out]
                        n282 = Array Max & Min(array=w354) -> (max value=w356:dbl, min value=w355:dbl)  [unwired: 2 out]
                        n283 = Equal?(x=w356, y=w355) -> (x = y?=w358:bool)
                        n284 = case shown="True" w358 {
                          tunnel: w357 -> [w361 w364]
                          tunnel: [w361 w362] -> w352
                          frame False {
                          }
                          frame True {
                            n285 = Delete From Array(array=w364, index (row)=0) -> (array with subset deleted=w362:dbl[][])  [unwired: 2 in, 1 out]
                          }
                        }
                        n286 = call "Load Final Data.vi"("measured data"=w352) -> ()  [unwired: 11 in]
                      }
                      frame True {
                      }
                    }
                  }
                  frame #1 {
                    n287 = case shown="False" w365 {
                      frame False {
                        n288 = local read "Data load indicator"() -> (w366:bool)
                        n289 = local write "Load Final Data"(FALSE ("Load Final Data")) -> ()
                        n290 = case shown="False" w366 {
                          frame False {
                            n291 = global read "Globals.vi" "Correction_num"() -> (w368:dbl)
                            n292 = Increment(x=w368) -> (x+1=w369:dbl)
                            n293 = global write "Globals.vi" "Correction_num"(w369) -> ()
                          }
                          frame True {
                          }
                        }
                      }
                      frame True {
                      }
                    }
                  }
                  frame #2 {
                    n294 = case shown="False" w370 {
                      frame False {
                        n295 = local read "Correction Factor K"() -> (w372:dbl)
                        n296 = call "Proportional Correction.vi"("Correction Factor K"=w372) -> ()  [unwired: 11 in]
                        "Data load indicator" <- TRUE
                      }
                      frame True {
                      }
                    }
                  }
                  frame #3 {
                    n297 = case shown="False" w373 {
                      frame False {
                        n298 = global read "Globals.vi" "transformed_error_all"() -> (w374:dbl[][])
                        n299 = Array Size(array=w374) -> (size(s)=w375:i32[])
                        n300 = Index Array(array=w375, index #1=1 ("index"), index #2=0 ("index")) -> (element #1=w381:i32, element #2=w379:i32)
                        n301 = Decrement(x=w381) -> (x-1=w382:i32)
                        n302 = Index Array(array=w374, index (col)=w382) -> (element=w377:dbl[])  [unwired: 1 in]
                        n303 = script code="normalized_err=norm(error)/sqrt(rows)"("error"=w377, "rows"=w379) -> ("normalized_err"=→"Normalized Error":dbl)  [unwired: 1 in, 1 out]
                      }
                      frame True {
                      }
                    }
                  }
                }
              }
            }
            n304 = Absolute Value(x="Spin Graph") -> (abs(x)=w270:dbl)
            n305 = Greater?(x=w270, y=0.001) -> (0:w268:bool)
            n306 = case shown="False" "Figure" {
              frame False {
              }
              frame True {
                n307 = script code="figure"() -> ()  [unwired: 1 in, 1 out]
                n308 = local write "Figure"(FALSE) -> ()
              }
            }
            n309 = case shown="True" w268 {
              tunnel: "Spin Graph" -> [_ w295]
              frame False {
              }
              frame True {
                n310 = property on="3D Surface" class="3D Surface (strict)"() -> ("Graph:View Longitude"=w296:sgl)  [unwired: 2 in, 2 out]
                n311 = Add(x=w296, y=w295) -> (x+y=w294:dbl)
                n312 = property on="3D Comet 3" class="3D Comet (strict)"("Graph:View Longitude"=w294) -> ()  [unwired: 2 in, 2 out]
                n313 = property on="3D Surface" class="3D Surface (strict)"("Graph:View Longitude"=w294) -> ()  [unwired: 2 in, 2 out]
              }
            }
            n314 = case shown="False" "Plot" {
              frame False {
              }
              frame True {
                n315 = global read "Globals.vi" "full_reference_data"() -> (w315:dbl[][])
                n316 = global read "Globals.vi" "initial_path"() -> (w313:dbl[][])
                n317 = global read "Globals.vi" "transformed data"() -> (w312:dbl[][])
                n318 = global read "Globals.vi" "correction_error"() -> (w311:dbl[][])
                n319 = global read "Globals.vi" "transformed_error_all"() -> (w310:dbl[][])
                n320 = global read "Globals.vi" "Plot_New_Path"() -> (w309:dbl[][])
                n321 = global read "Globals.vi" "avg_error_x"() -> (w307:dbl[][])
                n322 = global read "Globals.vi" "avg_error_y"() -> (w308:dbl[][])
                n323 = local write "Plot"(FALSE) -> ()
                n324 = script code="hold on\nswitch plot_type\n    case 0 % plot reference\n        plot3(full_reference_data(:,1), full_reference_data(:,2), full_reference_data(:,3))\n\n    case 1 % Plot Initial Command\n        plot3(initial_command(:,1),initial_command(:,2),initial_command(:,3))\n\n    case 2 % Plot transformed Data\n        plot3(transformed_data(:,1),transformed_data(:,2),transformed_data(:,3))\n\n    case 3\n        for index=1:min(size(transformed_error_all))\n            iteration_error(index)=norm(transformed_error_all(:,index))\n        end\n        plot(1:length(iteration_error),iteration_error,'o')\n        plot(1:length(iteration_error),iteration_error)\n    case 4 % Plot Error vs. Command\n        scatter(1:1:length(correction_error),correction_error);\n\n    case 5 % Plot Error Surface\n         [Xgrid,Ygrid] = meshgrid(1:3:254,1:3:254);\n         z_interp = griddata(full_reference_data(:,1),full_reference_data(:,2),transformed_error_all(:,correction_num),Xgrid,Ygrid);\n         zsurf = surf(Xgrid,Ygrid,z_interp);\n    case 6\n        plot3(current_correction(:,1),current_correction(:,2),current_correction(:,3))\n    case 7\n        plot(avg_error_x(:,1),avg_error_x(:,2),avg_error_y(:,1),avg_error_x(:,1))\n    otherwise\nend\nhold off"("plot_type"="Matlab Plot", "full_reference_data"=w315, "initial_command"=w313, "transformed_data"=w312, "correction_error"=w311, "transformed_error_all"=w310, "current_correction"=w309, "avg_error_x"=w307, "avg_error_y"=w308) -> ("??"=→"error out 2":errorcluster)  [unwired: 1 in]
                n325 = case shown="8" "Matlab Plot" {
                  frame 0, Default {
                  }
                  frame 8 {
                    n326 = call-poly <vilib>:"Read Delimited Spreadsheet.vi"("delimiter (\\t)"="," ("delimiter (\\t)")) -> ("all rows"=w323:dbl[][], "error out"=→"error out 5":errorcluster)  [unwired: 9 in, 4 out]
                    n327 = Index Array(array=w323, index (col) #1=0 ("disabled index (col)"), index (col) #2=1 ("index (col)"), index (col) #3=2 ("index (col)")) -> (element #1=w318:dbl[], element #2=w319:dbl[], element #3=w317:dbl[])  [unwired: 3 in]
                    n328 = script code="hold on\nplot3(x,y,z,format)\nhold off"("x"=w318, "y"=w319, "z"=w317, "format"="Graph Format Code") -> ()  [unwired: 1 in, 1 out]
                  }
                }
              }
            }
            n329 = local read "Data load indicator"() -> (w274:bool)
            n330 = case shown="True" "Upload Path" {
              frame False {
              }
              frame True {
                n331 = local write "Upload Path"(FALSE) -> ()
                n332 = call <vilib>:"FTP Put File.vi"("password"="", "user"="joseph", "remote path"="/hd0a/LAMP_FSW_IRB940/Programs/ISF/Modules/form_path.mod", "host"="r25dbristow.device.mst.edu") -> ("error out"=→"error out 4":errorcluster, "file error"=→"file error":errorcluster)  [unwired: 6 in]
              }
            }
            n333 = And(x="Save Correction", y=w274) -> (x .and. y?=w276:bool)
            n334 = case shown="True" w276 {
              frame False {
              }
              frame True {
                n335 = stacked-sequence {
                  frame #0 {
                    n336 = call-poly <vilib>:"Set Cursor.vi"("icon"=u16 2) -> ()  [unwired: 9 in, 2 out]
                  }
                  frame #1 {
                    n337 = call "Save Correction.vi"() -> ()  [unwired: 12 in]
                  }
                  frame #2 {
                    n338 = call-poly <vilib>:"Set Cursor.vi"("icon"=u16 0) -> ()  [unwired: 9 in, 2 out]
                    n339 = local write "Save Correction"(FALSE) -> ()
                    n340 = local write "Data load indicator"(FALSE) -> ()
                  }
                }
              }
            }
          }
        }
        n341 = case shown="False" "Close Figures" {
          frame False {
          }
          frame True {
            n342 = script code="close all"() -> ()  [unwired: 1 in, 1 out]
            n343 = local write "Close Figures"(FALSE ("Close Figures")) -> ()
          }
        }
        n344 = stacked-sequence {
          frame #0 {
            n345 = local read "Standby"() -> (w60:bool)
            n346 = And(x="Start Robot", y=w60) -> (x .and. y?=w59:bool)
            n347 = case shown="True" w59 {
              frame False {
              }
              frame True {
                n348 = local write "state"(1.0 ("state")) -> ()
                n349 = local write "Standby"(FALSE ("Start")) -> ()
              }
            }
            n350 = local write "Start Robot"(FALSE ("Start Robot")) -> ()
          }
          frame #1 {
            n351 = local read "VISA resource name out"() -> (w67:refnum<visa-resource-name>)
            n352 = property class="Instr"(reference=w67) -> (reference out=w72:refnum<visa-resource-name>, "Serial Settings:Number of Bytes at Serial Port"=w71:u32)  [unwired: 1 in, 1 out]
            n353 = VISA Read(VISA resource name=w72, byte count=w71) -> (read buffer=w68:string)  [unwired: 1 in, 3 out]
            n354 = Not Equal?(x=w68, y="") -> (x != y?=w70:bool)
            n355 = local read "state"() -> (w69:dbl)
            n356 = Select(t=w68, s=w70, f="waiting") -> (s? t:f=w66:string)
            n357 = case shown="1" w69 {
              tunnel: w67 -> [_ w83 _ w95 _]
              tunnel: w66 -> [_ w74 w84 _ _]
              frame 0, Default {
              }
              frame 1 {
                w81 = T5 32 items=["Flush Receive Buffer"=16, "Write Transmit Buffer to Device"=32, "Flush Receive Buffer (No I/O)"=64, "Flush Transmit Buffer"=128] ("Mask")
                n358 = local read "state"() -> (w76:dbl)
                n359 = Equal?(x=w74, y="s") -> (x = y?=w77:bool)
                n360 = VISA Write(VISA resource name=w83, write buffer="00001") -> (VISA resource name out=w82:refnum<visa-resource-name>)  [unwired: 1 in, 2 out]
                n361 = Select(t=2.0, s=w77, f=w76) -> (s? t:f=w75:dbl)
                n362 = local write "state"(w75) -> ()
                n363 = property on="Standby" class="Bool (strict)"("Blinking"=FALSE) -> ()  [unwired: 2 in, 2 out]
                n364 = VISA Flush I/O Buffer(VISA resource name=w82, mask (16)=w81) -> ()  [unwired: 1 in, 2 out]
              }
              frame 2 {
                n365 = local read "state"() -> (w85:dbl)
                n366 = Equal?(x=w84, y="e") -> (x = y?=w86:bool)
                n367 = Select(t=4.0, s=w86, f=w85) -> (s? t:f=w87:dbl)
                n368 = local write "state"(w87) -> ()
              }
              frame 3 {
                w93 = T5 32 items=["Flush Receive Buffer"=16, "Write Transmit Buffer to Device"=32, "Flush Receive Buffer (No I/O)"=64, "Flush Transmit Buffer"=128] ("Mask")
                n369 = VISA Write(VISA resource name=w95, write buffer="00000") -> (VISA resource name out=w94:refnum<visa-resource-name>)  [unwired: 1 in, 2 out]
                n370 = property on="Standby" class="Bool (strict)"("BoolText.Text"="STOPPED" ("Boolean Text.Text"), "Blinking"=TRUE) -> ()  [unwired: 2 in, 2 out]
                n371 = VISA Flush I/O Buffer(VISA resource name=w94, mask (16)=w93) -> ()  [unwired: 1 in, 2 out]
              }
              frame 4 {
                n372 = local read "state"() -> (w98:dbl)
                n373 = Select(t=3.0, s="Stop Robot", f=w98) -> (s? t:f=w97:dbl)
                n374 = local write "state"(w97) -> ()
                "Standby" <- TRUE
              }
            }
          }
        }
        n375 = case shown="False" "Open Webcam" {
          frame False {
          }
          frame True {
            n376 = local write "Open Webcam"(FALSE) -> ()
            n377 = Current VI's Path() -> (path=w104:path)
            n378 = Path to Array of Strings(0:w104) -> (2:w105:string[])  [unwired: 1 out]
            n379 = Array Size(array=w105) -> (size(s)=w102:i32)
            n380 = Decrement(x=w102) -> (x-1=w101:i32)
            n381 = Delete From Array(array=w105, index=w101) -> (array with subset deleted=w106:string[])  [unwired: 1 in, 1 out]
            n382 = Array of Strings to Path(0:w106) -> (2:w107:path)  [unwired: 1 in]
            n383 = call <vilib>:"System Exec.vi"("working directory"=w107, "command line"="cmd /c Webcam.vi") -> ()  [unwired: 6 in, 4 out]
          }
        }
      }
      n384 = while {
        stop <- w50 stop-if-true
        n385 = event shown="[0] Timeout" {
          selector: _ -> [_ _]
          dyn-events: _ -> [_ _]
          timeout: 500 -> [_ _]
          event Timeout {
            n386 = event-data() -> ()  [unwired: 1 in, 3 out]
          }
          event "Correction Factor K": Value Change {
            n387 = event-data() -> ()  [unwired: 1 in, 6 out]
            n388 = local read "Data load indicator"() -> (w51:bool)
            n389 = case shown="True" w51 {
              frame False {
              }
              frame True {
                n390 = local read "Correction Factor K"() -> (w52:dbl)
                n391 = call "Proportional Correction.vi"("Correction Factor K"=w52) -> ()  [unwired: 11 in]
              }
            }
          }
        }
        n392 = local read "stop"() -> (w50:bool)
      }
    }
  }
